vi "Slave on RT Target.vi"() -> ()   [LabVIEW 2021]
doc: "Demonstrates how to use Modbus functions on RT to create a Modbus slave listening to a specific TCP port. It updates the input registers on the virtual device with an auto-incremental value and then read it out to an array. It will also get the count of masters connected to this slave. The value read out and the count of masters is updated every 1 second automatically."
uses:
  Modbus_v121c/API/Wrapper/Create TCP Slave.vi
  Modbus_v121c/API/Slave/Modbus Slave.lvclass
  Modbus_v121c/API/Wrapper/API Main.lvlib
panel:
  in  "milliseconds to wait":u32=1
  out "Number of Masters":u32
  out "Input Registers Read":u16[](array[numeric])
  in  "Auto Write? (T)":bool=TRUE
  in  "Stop":bool
  # "Overview: Demonstrates the use of the Modbus Slave VIs on a LabVIEW Real-Time target to create a Modbus slave, use the Modbus slave to read and write the values of input registers on this Modbus slave, and use the Modbus slave to read the number of Modbus masters connected to this Modbus slave.\nRequirements: LabVIEW Real-Time Module\nInstructions:\n1. In the Project Explorer Window, specify an IP address for the RT target.\n2. Ensure Port 502 is not in use.\n3. Run the VI.\n4. Click Stop to stop the VI.\nNote: You can set Auto Write? to FALSE if you do not want to write values to input registers every one second."
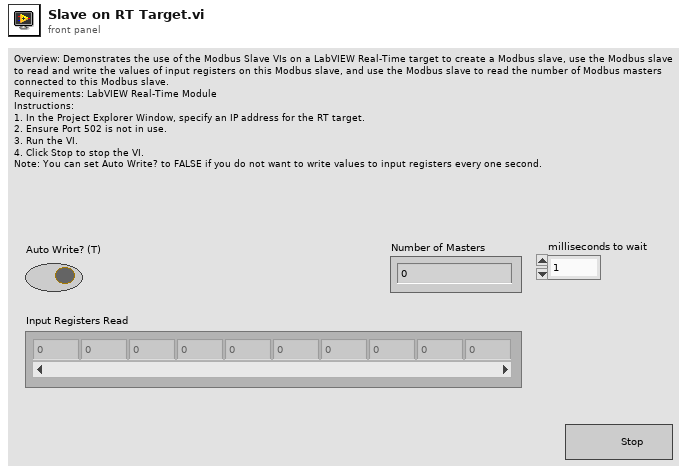
[diagram p1: front panel]
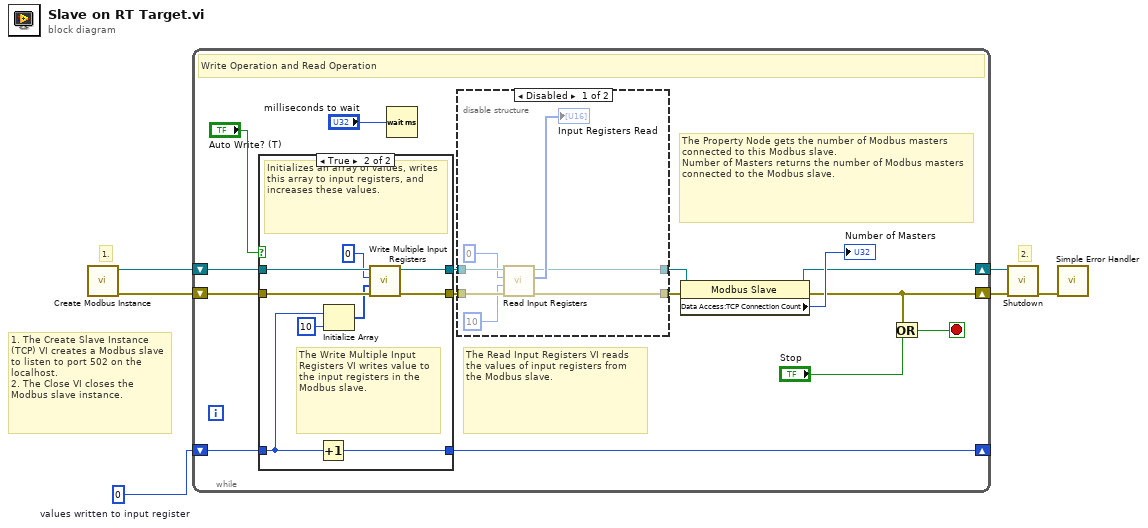
[diagram p0: block diagram]
diagram:
  w2 = u16 0  # values written to input register
  # "2."
  # "1."
  # "1. The Create Slave Instance (TCP) VI creates a Modbus slave to listen to port 502 on the localhost.\n2. The Close VI closes the Modbus slave instance."
  n1 = call-poly "Create Modbus Instance.vi"() -> ("error out"=w5:errorcluster, "TCP slave instance"=w6:refnum<class "Modbus Slave.lvclass">)  [unwired: 10 in]
  n2 = while {
    shift-right: [w11] -> w3
    shift-left: w6 -> [w18]
    shift-right: [w9] -> w4
    shift-left: w5 -> [w17]
    shift-right: [w7] -> _
    shift-left: w2 -> [w8]
    stop <- w10 stop-if-true
    # "The Property Node gets the number of Modbus masters connected to this Modbus slave.\nNumber of Masters returns the number of Modbus masters connected to the Modbus slave."
    # "The Read Input Registers VI reads the values of input registers from the Modbus slave."
    # "Write Operation and Read Operation"
    n3 = case shown="True" "Auto Write? (T)" {
      tunnel: w18 -> [w33 w42]
      tunnel: [w33 w40] -> w16
      tunnel: w17 -> [w32 w39]
      tunnel: [w32 w38] -> w15
      tunnel: w8 -> [w31 w34]
      tunnel: [w31 w35] -> w7
      frame False {
      }
      frame True {
        # "The Write Multiple Input Registers VI writes value to the input registers in the Modbus slave."
        # "Initializes an array of values, writes this array to input registers, and increases these values."
        n4 = Increment(x=w34) -> (x+1=w35:u16)
        n5 = Initialize Array(w34, 10 ("dimension size")) -> (w36:u16[])
        n6 = call-dynamic "Write Multiple Input Registers.vi"("error in (no error)"=w39, "input register values"=w36, "starting address"=u16 0, "Modbus slave in"=w42) -> ("error out"=w38:errorcluster, "Modbus slave out"=w40:refnum<class "Modbus Slave.lvclass">)  [unwired: 6 in]
      }
    }
    n7 = Wait (ms)(milliseconds to wait="milliseconds to wait") -> ()  [unwired: 1 out]
    n8 = disable-structure shown="Disabled" {
      disable-tunnel: w16 -> [w28 w30]
      disable-tunnel: w15 -> [w27 w29]
      disable-tunnel: [w23 w30] -> w14
      disable-tunnel: [w22 w29] -> w13
      frame Disabled {
        n9 = call-dynamic "Read Input Registers.vi"("error in (no error)"=w27, "number of input registers"=u16 10 ("number of inputs"), "starting address"=u16 0, "Modbus slave in"=w28) -> ("error out"=w22:errorcluster, "register values"=→"Input Registers Read":u16[], "Modbus slave out"=w23:refnum<class "Modbus Slave.lvclass">)  [unwired: 5 in]
      }
      frame Enabled {
      }
    }
    n10 = property class="Modbus Slave"(reference=w14, error in=w13) -> (reference out=w11:refnum<class "Modbus Slave.lvclass">, error out=w9:errorcluster, "Data Access:TCP Connection Count"=→"Number of Masters":u32)
    n11 = Or(x=w9, y="Stop") -> (x .or. y?=w10:bool)
  }
  n12 = call-dynamic "Shutdown.vi"("error in (no error)"=w4, "Modbus slave in"=w3) -> ("error out"=w1:errorcluster)  [unwired: 9 in]
  n13 = call <vilib>:"Simple Error Handler.vi"("error in (no error)"=w1) -> ()  [unwired: 4 in, 5 out]
